vi "Read Current Step.vi"(8 "error in (no error)":errorcluster, 11 "Double Scanner in":refnum<class "Double Scanner.lvclass">) -> (0 "error out":errorcluster, 1 "Current Position Array":dbl[](array[numeric]), 2 "Current step":u32, 3 "Double Scanner out":refnum<class "Double Scanner.lvclass">, 4 "Total steps":i32)   [LabVIEW 2015, in "Double Scanner.lvclass"]
uses:
  Double Scanner.lvclass
  Scanner/Scanner.lvclass
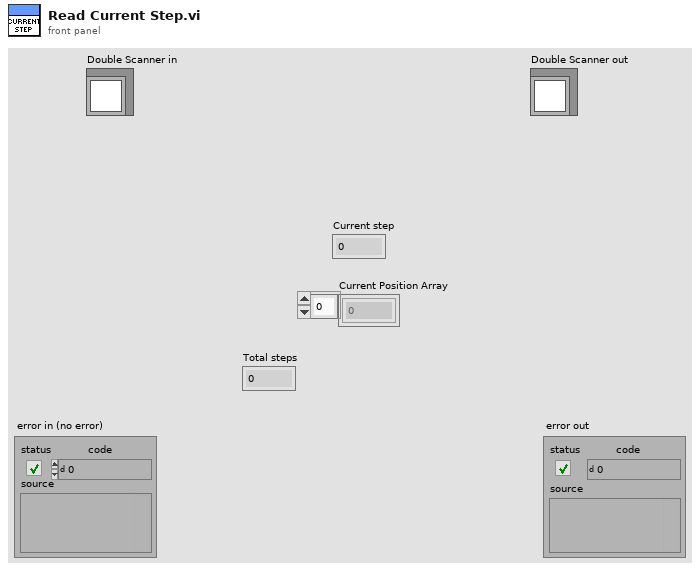
[diagram p1: front panel]
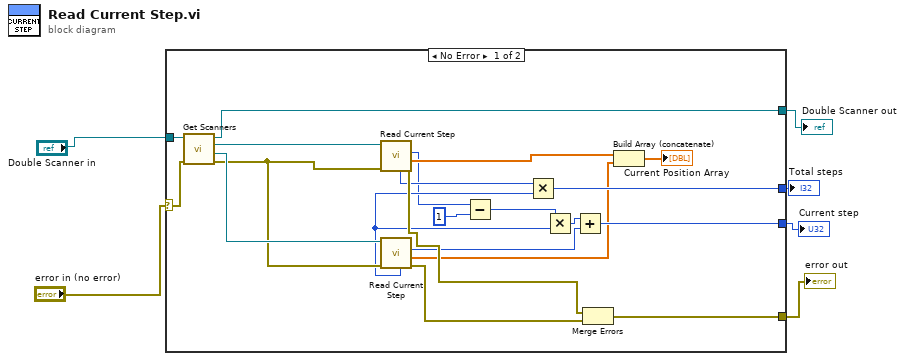
[diagram p0: block diagram]
diagram:
  n1 = case shown="No Error" "error in (no error)" {
    selector: "error in (no error)" -> [w22 w29]
    tunnel: "Double Scanner in" -> [w23 w28]
    tunnel: [w21 w29] -> w4
    tunnel: [w20 _] -> w3
    tunnel: [w19 _] -> w2
    tunnel: [w18 w28] -> w1
    frame No Error {
      n2 = call-dynamic "Get Scanners.vi"("error in (no error)"=w22, "Double Scanner in"=w23) -> ("error out"=w13:errorcluster, "Scanner 2 out"=w14:refnum<class "Scanner.lvclass">, "Scanner 1 out"=w12:refnum<class "Scanner.lvclass">, "Double Scanner out"=w18:refnum<class "Double Scanner.lvclass">)  [unwired: 6 in]
      n3 = call-dynamic "Read Current Step.vi"("error in (no error)"=w13, "Scanner.lvclass in"=w12) -> ("error out"=w26:errorcluster, "Current Position Array"=w17:dbl[], "Current Step"=w9:u32, "Total Steps"=w11:i32)  [unwired: 5 in, 1 out]
      n4 = call-dynamic "Read Current Step.vi"("error in (no error)"=w13, "Scanner.lvclass in"=w14) -> ("error out"=w27:errorcluster, "Current Position Array"=w16:dbl[], "Current Step"=w24:u32, "Total Steps"=w10:i32)  [unwired: 5 in, 1 out]
      n5 = Subtract(x=w9, y=u32 1) -> (x-y=w7:u32)
      n6 = Multiply(x=w11, y=w10) -> (x*y=w20:i32)
      n7 = Multiply(x=w7, y=w10) -> (x*y=w25:u32)
      n8 = Add(x=w25, y=w24) -> (x+y=w19:u32)
      n9 = Merge Errors(w26, w27) -> (w21:errorcluster)
      n10 = Build Array (concatenate)(w17, w16) -> (→"Current Position Array":dbl[])
    }
    frame Error {
    }
  }
  "Total steps" <- w3
  "Current step" <- w2
  "error out" <- w4
  "Double Scanner out" <- w1
